vi "UpdateSweepStatistics.vi"(6 "sweep complete":bool[](array[boolean]), 8 "error in (no error)":errorcluster, 9 "current sweep frequencies":dbl[](array[numeric]), 10 "sweep times":dbl[](array[numeric]), 11 "channels":string[](array[string])) -> (0 "error out":errorcluster)   [LabVIEW 2017, in "EmsaAcquisition.lvlib"]
uses:
  <vilib>/addons/InsightCM/Devices/Shared/Emsa/EmsaAcquisition/EmsaAcquisition.lvlib
  InsightCM/Devices/WebServices/Emsa/accessors/SweepStats.ctl
  InsightCM/Devices/WebServices/Emsa/accessors/EmsaWebServiceAccessors.lvlib
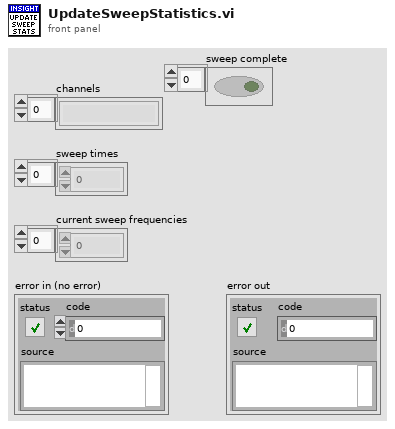
[diagram p1: front panel]
types:
  T1 = typedef "EmsaWebServiceAccessors.lvlib/SweepStats.ctl" = cluster{"Channel":string, "Sweep Time(min)":dbl, "Current Frequency(Hz)":dbl, "Max Sweep Time(min)":dbl, "Completed Sweep":bool}
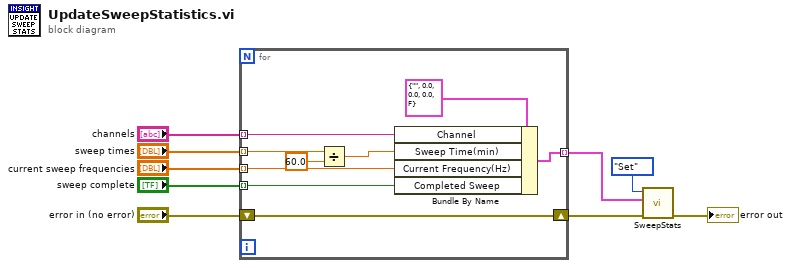
[diagram p0: block diagram]
diagram:
  n1 = for {
    tunnel: "channels" -> [w17] mode=indexing
    tunnel: "sweep times" -> [w13] mode=indexing
    tunnel: "current sweep frequencies" -> [w16] mode=indexing
    shift-right: [w15] -> w5
    shift-left: "error in (no error)" -> [w15]
    tunnel: [w14] -> w3 mode=indexing
    tunnel: "sweep complete" -> [w10] mode=indexing
    n2 = Divide(x=w13, y=60.0) -> (x/y=w11:dbl)
    n3 = Bundle By Name(cluster=T1 {"Channel"="", "Sweep Time(min)"=0.0, "Current Frequency(Hz)"=0.0, "Max Sweep Time(min)"=0.0, "Completed Sweep"=FALSE} ("Sweep Stats"), "Channel"=w17, "Sweep Time(min)"=w11, "Current Frequency(Hz)"=w16, "Completed Sweep"=w10) -> (w14:T1)
  }
  n4 = call "SweepStats.vi"("error in (no error)"=w5, "Sweep Stats"=w3, "Action"=enum16{"Get", "Set"}."Set") -> ("error out"=→"error out":errorcluster)  [unwired: 7 in, 1 out]
